vi "F to C (SubVI).vi"(8 "Boolean":bool, 11 "Temperature (F)":dbl) -> (3 "Numeric":dbl)   [LabVIEW 2017]
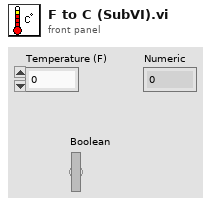
[diagram p1: front panel]
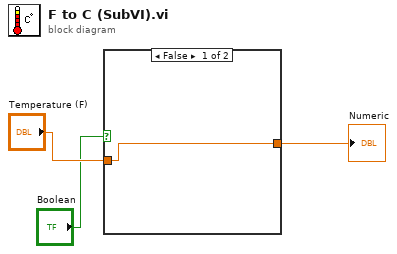
[diagram p0: block diagram]
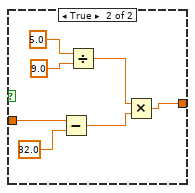
[diagram p2: hidden frame]
diagram:
  n1 = case shown="False" "Boolean" {
    tunnel: [w4 w11] -> w3
    tunnel: "Temperature (F)" -> [w4 w5]
    frame False {
    }
    frame True {
      n2 = Subtract(x=w5, y=32.0) -> (x-y=w6:dbl)
      n3 = Divide(x=5.0, y=9.0) -> (x/y=w7:dbl)
      n4 = Multiply(x=w7, y=w6) -> (x*y=w11:dbl)
    }
  }
  "Numeric" <- w3
